vi "Run VI Transparently.vi"(8 "error in (no error)":errorcluster, 11 "VI Ref In":refnum<vi>) -> (0 "error out":errorcluster, 3 "VI Ref Out":refnum<vi>)   [LabVIEW 2016, in "SLL Splash Screen.lvlib"]
uses:
  SLL Splash Screen.lvlib
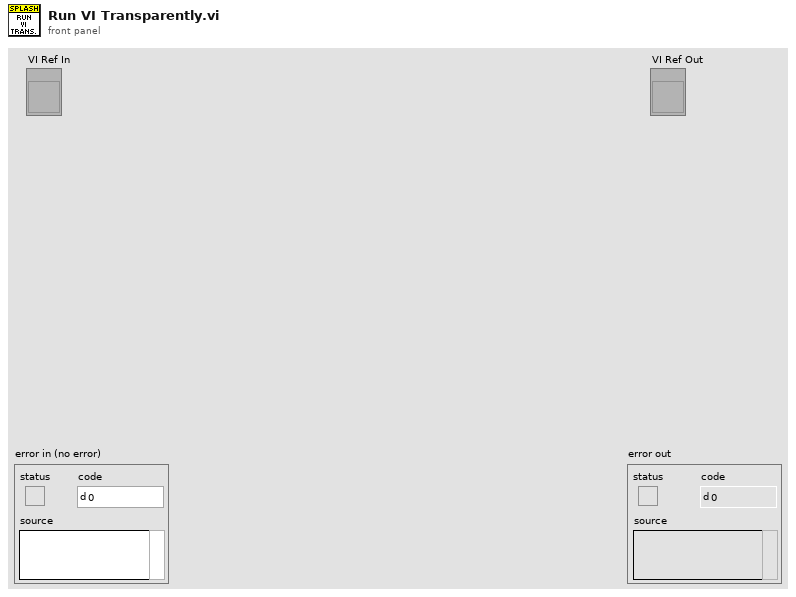
[diagram p1: front panel]
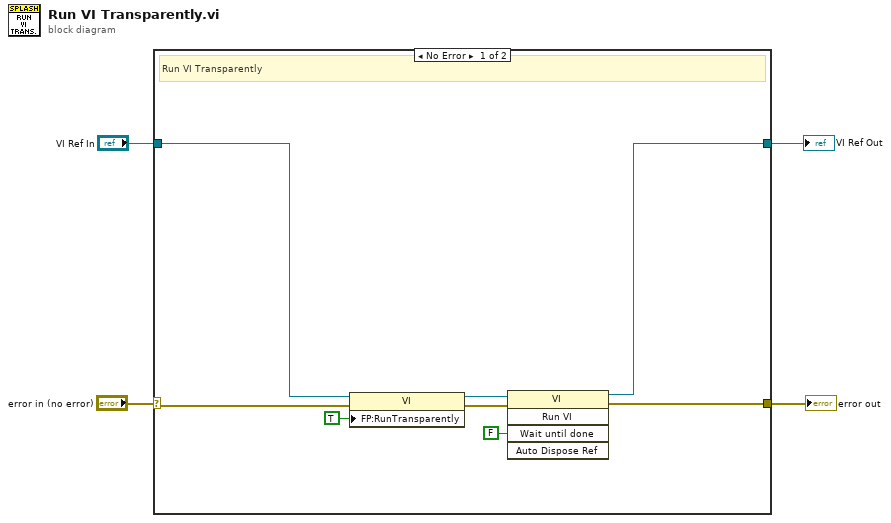
[diagram p0: block diagram]
diagram:
  n1 = case shown="No Error" "error in (no error)" {
    selector: "error in (no error)" -> [w8 w14]
    tunnel: [w7 w14] -> w3
    tunnel: "VI Ref In" -> [w6 w13]
    tunnel: [w5 w13] -> w1
    frame No Error {
      # "Run VI Transparently"
      n2 = property class="VI"(reference=w6, error in=w8, "FP:RunTransparently"=TRUE ("Front Panel Window:Run VI Transparently")) -> (reference out=w10:refnum<vi>, error out=w9:errorcluster)
      n3 = invoke class="VI" method="Run VI"(reference=w10, error in=w9, "Wait until done"=FALSE ("Wait Until Done")) -> (reference out=w5:refnum<vi>, error out=w7:errorcluster)  [unwired: 2 in, 3 out]
    }
    frame Error {
    }
  }
  "error out" <- w3
  "VI Ref Out" <- w1
